vi "Init Tx Header.vi"(8 "error in (no error)":errorcluster, 11 "Tx Loop Data":T1) -> (0 "error out":errorcluster, 3 "Tx Loop Data out":T1)   [LabVIEW 2016, in "UDP-Custom-Device Engine.lvlib"]
uses:
  UDP-Custom-Device Engine.lvlib
  Tx Loop Data.ctl
  <vilib>/NI Veristand/VeriStand Data/Library/Byte Buffer/Byte Buffer.lvclass
  <vilib>/NI/NIVS Inline Async API/_Data Access Engine/Data Access Engine/Types/Read.DVR.ctl
  <vilib>/NI/NIVS Inline Async API/_Data Access Engine/Access Type Classes/Read/Read.lvclass
  <vilib>/NI Veristand/VeriStand Data/Library/Typedefs/Typedefs.Data Types.ctl
  Data Conversion Config.ctl
  <vilib>/NI Veristand/VeriStand Data/Library/Byte Buffer/Byte Buffer.Mapping.ctl
  Shared/Header Details.ctl
  <vilib>/NI/NIVS Inline Async API/_Data Access Engine/Data Access Engine/Data Access Engine.lvclass
  <vilib>/NI Veristand/VeriStand Data/Library/VeriStand Data.lvlib
  Shared/UDP-Custom-Device Shared.lvlib
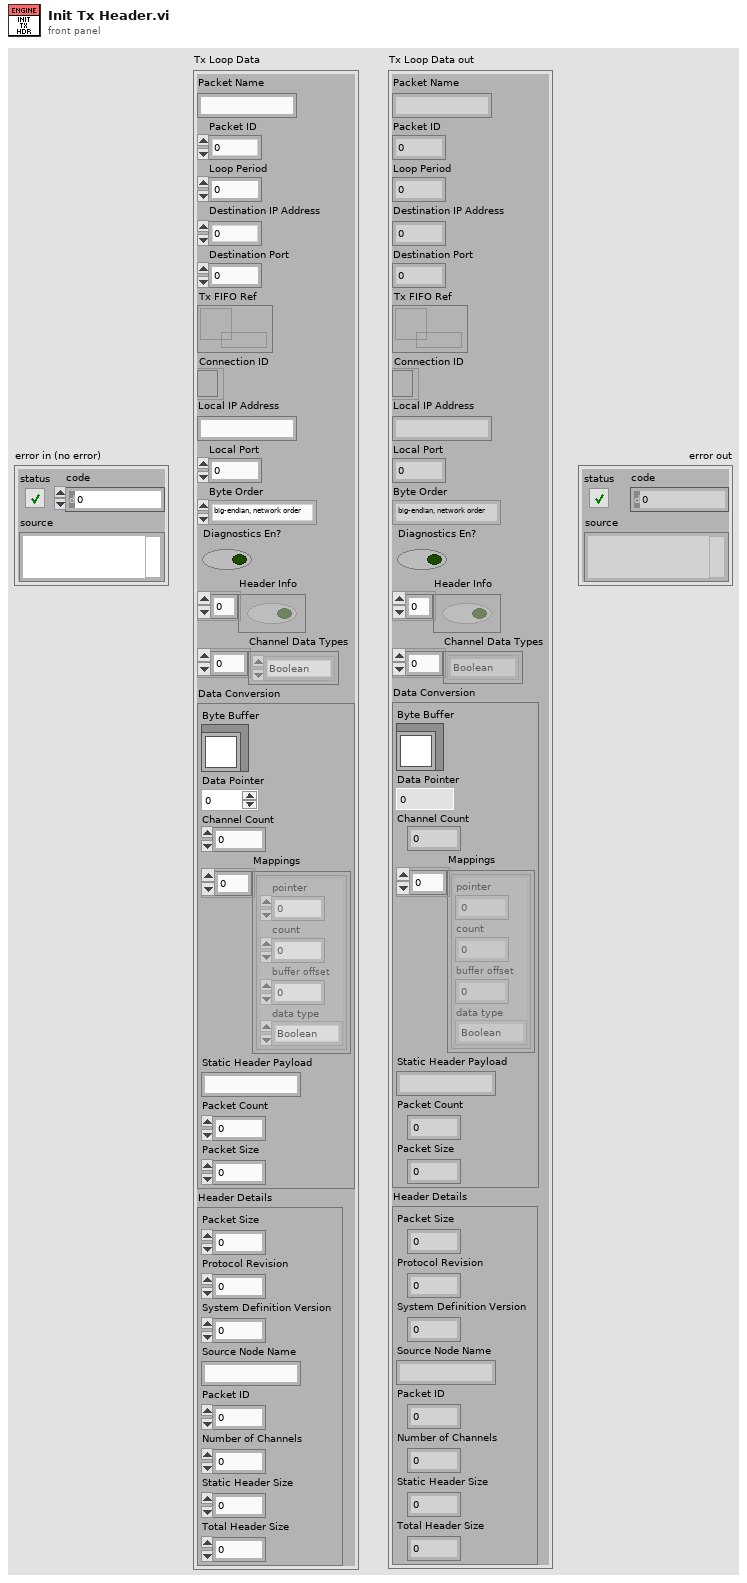
[diagram p1: front panel]
types:
  T1 = typedef "UDP-Custom-Device Engine.lvlib/Tx Loop Data.ctl" = cluster{"Packet Name":string, "Packet ID":i32, "Loop Period":u32, "Destination IP Address":u32, "Destination Port":u16, "Tx FIFO Ref":T2, "Connection ID":refnum<k16>, "Local IP Address":string, "Local Port":i32, "Byte Order":enum16{"big-endian, network order", "native, host order", "little-endian"}, "Diagnostics En?":bool, "Header Info":bool[], "Channel Data Types":T3[], "Data Conversion":T4, "Header Details":T6}
  T2 = typedef "Data Access Engine.lvlib/Data Access Engine.lvclass/Read.DVR.ctl" = refnum<data-value>
  T3 = typedef "VeriStand Data.lvlib/Typedefs.Data Types.ctl" = enum16{"Boolean", "Single", "Double", "I8", "I16", "I32", "I64", "U8", "U16", "U32", "U64"}
  T4 = typedef "UDP-Custom-Device Engine.lvlib/Data Conversion Config.ctl" = cluster{"Byte Buffer":refnum<class "Byte Buffer.lvclass">, "Data Pointer":u64, "Channel Count":i32, "Mappings":T5[], "Static Header Payload":string, "Packet Count":dbl, "Packet Size":i32}
  T5 = typedef "VeriStand Data.lvlib/Byte Buffer.lvclass/Byte Buffer.Mapping.ctl" = cluster{"pointer":u64, "count":i32, "buffer offset":i32, "data type":T3}
  T6 = typedef "UDP-Custom-Device Shared.lvlib/Header Details.ctl" = cluster{"Packet Size":u16, "Protocol Revision":u8, "System Definition Version":u16, "Source Node Name":string, "Packet ID":u32, "Number of Channels":u32, "Static Header Size":u16, "Total Header Size":u16}
  T7 = enum16{"big-endian, network order", "native, host order", "little-endian"}
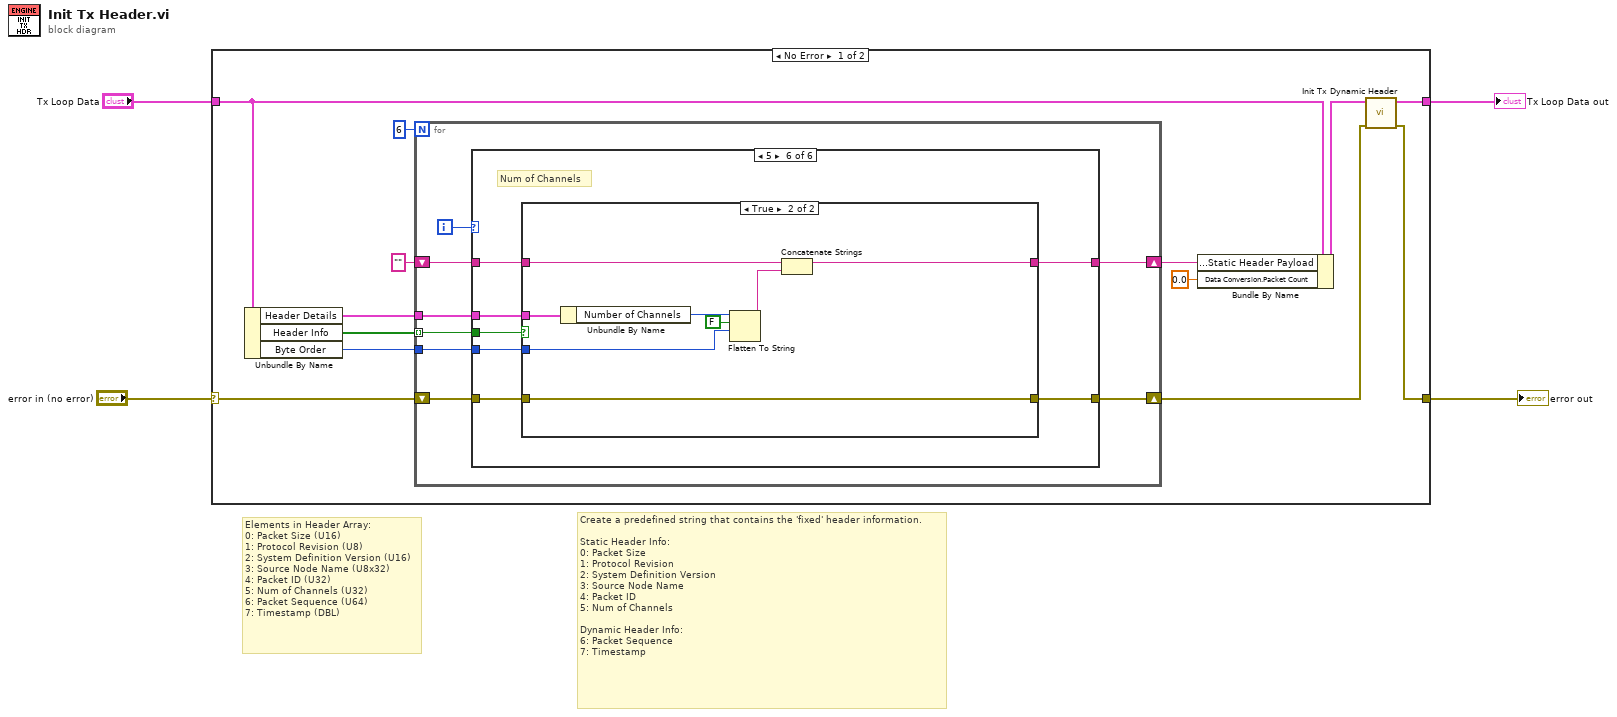
[diagram p0: block diagram]
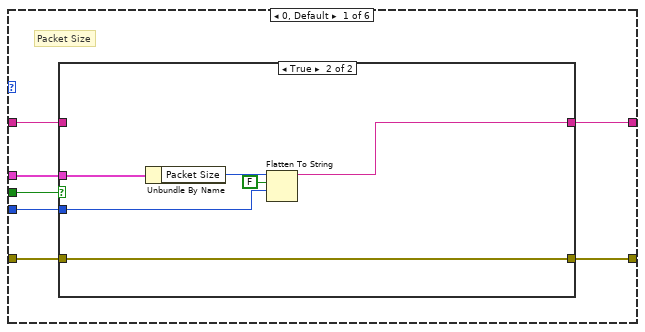
[diagram p2: hidden frame]
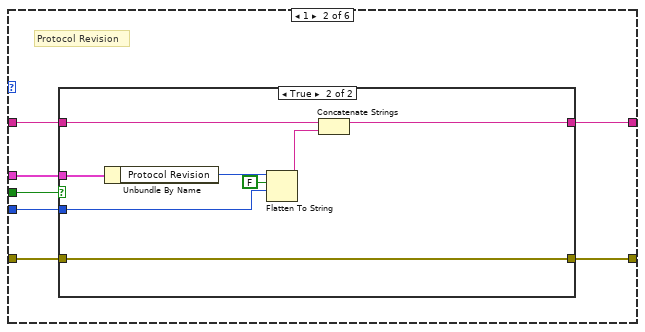
[diagram p4: hidden frame]
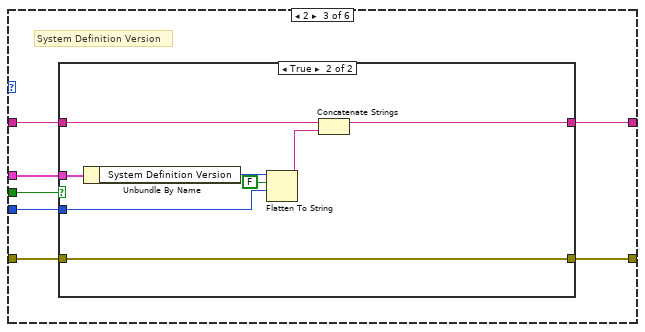
[diagram p6: hidden frame]
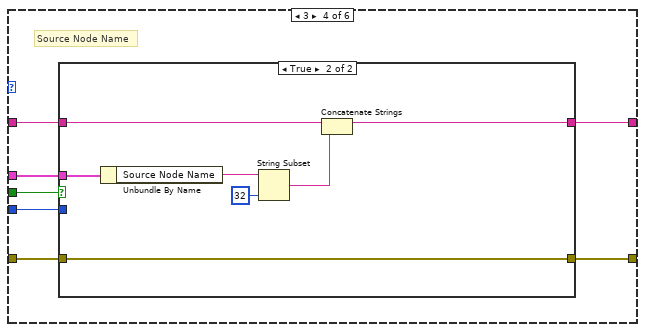
[diagram p8: hidden frame]
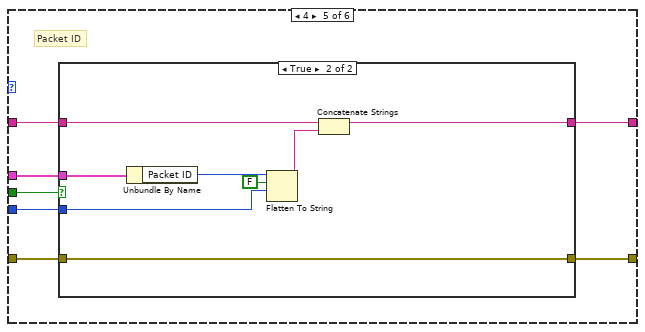
[diagram p10: hidden frame]
diagram:
  # "Create a predefined string that contains the 'fixed' header information.\n\nStatic Header Info:\n0: Packet Size\n1: Protocol Revision\n2: System Definition Version\n3: Source Node Name\n4: Packet ID\n5: Num of Channels\n\nDynamic Header Info:\n6: Packet Sequence\n7: Timestamp"
  # "Elements in Header Array:\n0: Packet Size (U16)\n1: Protocol Revision (U8)\n2: System Definition Version (U16)\n3: Source Node Name (U8x32)\n4: Packet ID (U32)\n5: Num of Channels (U32)\n6: Packet Sequence (U64)\n7: Timestamp (DBL)"
  n1 = case shown="No Error" "error in (no error)" {
    selector: "error in (no error)" -> [w17 w126]
    tunnel: [w5 w126] -> w3
    tunnel: "Tx Loop Data" -> [w9 w125]
    tunnel: [w7 w125] -> w1
    frame No Error {
      n2 = Unbundle By Name(w9) -> ("Header Details"=w14:T6, "Header Info"=w16:bool[], "Byte Order"=w13:T7)
      n3 = for {
        N: 6 -> [_]
        shift-right: [w24] -> w6
        shift-left: w17 -> [w25]
        tunnel: w16 -> [w21] mode=indexing
        tunnel: w14 -> [w22]
        tunnel: w13 -> [w20]
        shift-right: [w19] -> w11
        shift-left: "" ("data string") -> [w18]
        i -> [w23]
        n4 = case shown="5" w23 {
          tunnel: w25 -> [w31 w46 w63 w80 w96 w113]
          tunnel: [w32 w47 w64 w81 w97 w114] -> w24
          tunnel: w22 -> [w29 w44 w61 w78 w94 w111]
          tunnel: w21 -> [w30 w45 w62 w79 w95 w112]
          tunnel: w20 -> [w28 w43 w60 w77 w93 w110]
          tunnel: [w27 w42 w59 w76 w92 w109] -> w19
          tunnel: w18 -> [w26 w41 w58 w75 w91 w108]
          frame 0, Default {
            # "Packet Size"
            n5 = case shown="True" w30 {
              tunnel: [w34 w40] -> w32
              tunnel: w31 -> [w34 w40]
              tunnel: w29 -> [_ w39]
              tunnel: w28 -> [_ w37]
              tunnel: [w33 w35] -> w27
              tunnel: w26 -> [w33 _]
              frame False {
              }
              frame True {
                n6 = Unbundle By Name(w39) -> ("Packet Size"=w38:u16)
                n7 = Flatten To String(anything=w38, prepend array or string size? (T)=FALSE, byte order (0:big-endian, network order)=w37) -> (data string=w35:string)  [unwired: 1 in, 2 out]
              }
            }
          }
          frame 1 {
            # "Protocol Revision"
            n8 = case shown="True" w45 {
              tunnel: [w49 w57] -> w47
              tunnel: w46 -> [w49 w57]
              tunnel: w44 -> [_ w56]
              tunnel: w43 -> [_ w54]
              tunnel: [w48 w50] -> w42
              tunnel: w41 -> [w48 w52]
              frame False {
              }
              frame True {
                n9 = Unbundle By Name(w56) -> ("Protocol Revision"=w55:u8)
                n10 = Flatten To String(anything=w55, prepend array or string size? (T)=FALSE, byte order (0:big-endian, network order)=w54) -> (data string=w51:string)  [unwired: 1 in, 2 out]
                n11 = Concatenate Strings(w52, w51) -> (w50:string)
              }
            }
          }
          frame 2 {
            # "System Definition Version"
            n12 = case shown="True" w62 {
              tunnel: [w66 w74] -> w64
              tunnel: w63 -> [w66 w74]
              tunnel: w61 -> [_ w73]
              tunnel: w60 -> [_ w71]
              tunnel: [w65 w67] -> w59
              tunnel: w58 -> [w65 w69]
              frame False {
              }
              frame True {
                n13 = Unbundle By Name(w73) -> ("System Definition Version"=w72:u16)
                n14 = Flatten To String(anything=w72, prepend array or string size? (T)=FALSE, byte order (0:big-endian, network order)=w71) -> (data string=w68:string)  [unwired: 1 in, 2 out]
                n15 = Concatenate Strings(w69, w68) -> (w67:string)
              }
            }
          }
          frame 3 {
            # "Source Node Name"
            n16 = case shown="True" w79 {
              tunnel: [w83 w90] -> w81
              tunnel: w80 -> [w83 w90]
              tunnel: w78 -> [_ w89]
              tunnel: w77 -> [_ _]
              tunnel: [w82 w87] -> w76
              tunnel: w75 -> [w82 w88]
              frame False {
              }
              frame True {
                n17 = Unbundle By Name(w89) -> ("Source Node Name"=w86:string)
                n18 = String Subset(string=w86, length (rest)=32 ("length (rest)")) -> (substring=w84:string)  [unwired: 1 in]
                n19 = Concatenate Strings(w88, w84) -> (w87:string)
              }
            }
          }
          frame 4 {
            # "Packet ID"
            n20 = case shown="True" w95 {
              tunnel: [w99 w107] -> w97
              tunnel: w96 -> [w99 w107]
              tunnel: w94 -> [_ w106]
              tunnel: w93 -> [_ w104]
              tunnel: [w98 w100] -> w92
              tunnel: w91 -> [w98 w102]
              frame False {
              }
              frame True {
                n21 = Unbundle By Name(w106) -> ("Packet ID"=w105:u32)
                n22 = Flatten To String(anything=w105, prepend array or string size? (T)=FALSE, byte order (0:big-endian, network order)=w104) -> (data string=w101:string)  [unwired: 1 in, 2 out]
                n23 = Concatenate Strings(w102, w101) -> (w100:string)
              }
            }
          }
          frame 5 {
            # "Num of Channels"
            n24 = case shown="True" w112 {
              tunnel: [w116 w124] -> w114
              tunnel: w113 -> [w116 w124]
              tunnel: w111 -> [_ w123]
              tunnel: w110 -> [_ w121]
              tunnel: [w115 w117] -> w109
              tunnel: w108 -> [w115 w119]
              frame False {
              }
              frame True {
                n25 = Unbundle By Name(w123) -> ("Number of Channels"=w122:u32)
                n26 = Flatten To String(anything=w122, prepend array or string size? (T)=FALSE, byte order (0:big-endian, network order)=w121) -> (data string=w118:string)  [unwired: 1 in, 2 out]
                n27 = Concatenate Strings(w119, w118) -> (w117:string)
              }
            }
          }
        }
      }
      n28 = Bundle By Name(cluster=w9, "Data Conversion.Static Header Payload"=w11, "Data Conversion.Packet Count"=0.0) -> (w8:T1)
      n29 = call "Init Tx Dynamic Header.vi"("error in (no error)"=w6, "Tx Loop Data"=w8) -> ("error out"=w5:errorcluster, "Tx Loop Data out"=w7:T1)  [unwired: 8 in]
    }
    frame Error {
    }
  }
  "error out" <- w3
  "Tx Loop Data out" <- w1
